vi "Main.vi"() -> ()   [LabVIEW 2017]
doc: "Use this template to build a simple state machine design pattern. Each state executes code and determines which state to transition to."
uses:
  Controls/Database_Array.ctl
  Controls/Encoding.ctl
  <userlib>/_OpenG.lib/array/array.llb/Search 1D Array (I32)__ogtk.vi
  <userlib>/_OpenG.lib/array/array.llb/Index 1D Array Elements (Variant)__ogtk.vi
  Controls/State.ctl
  Controls/Data.ctl
panel:
  out "Error (out)":errorcluster
  out "Parameter Array":T1[](array[typedef])
  out "HW File":string
  out "Param File":string
  in  "Core ID":i32=-1
  in  "Core Name":string="CoreName"
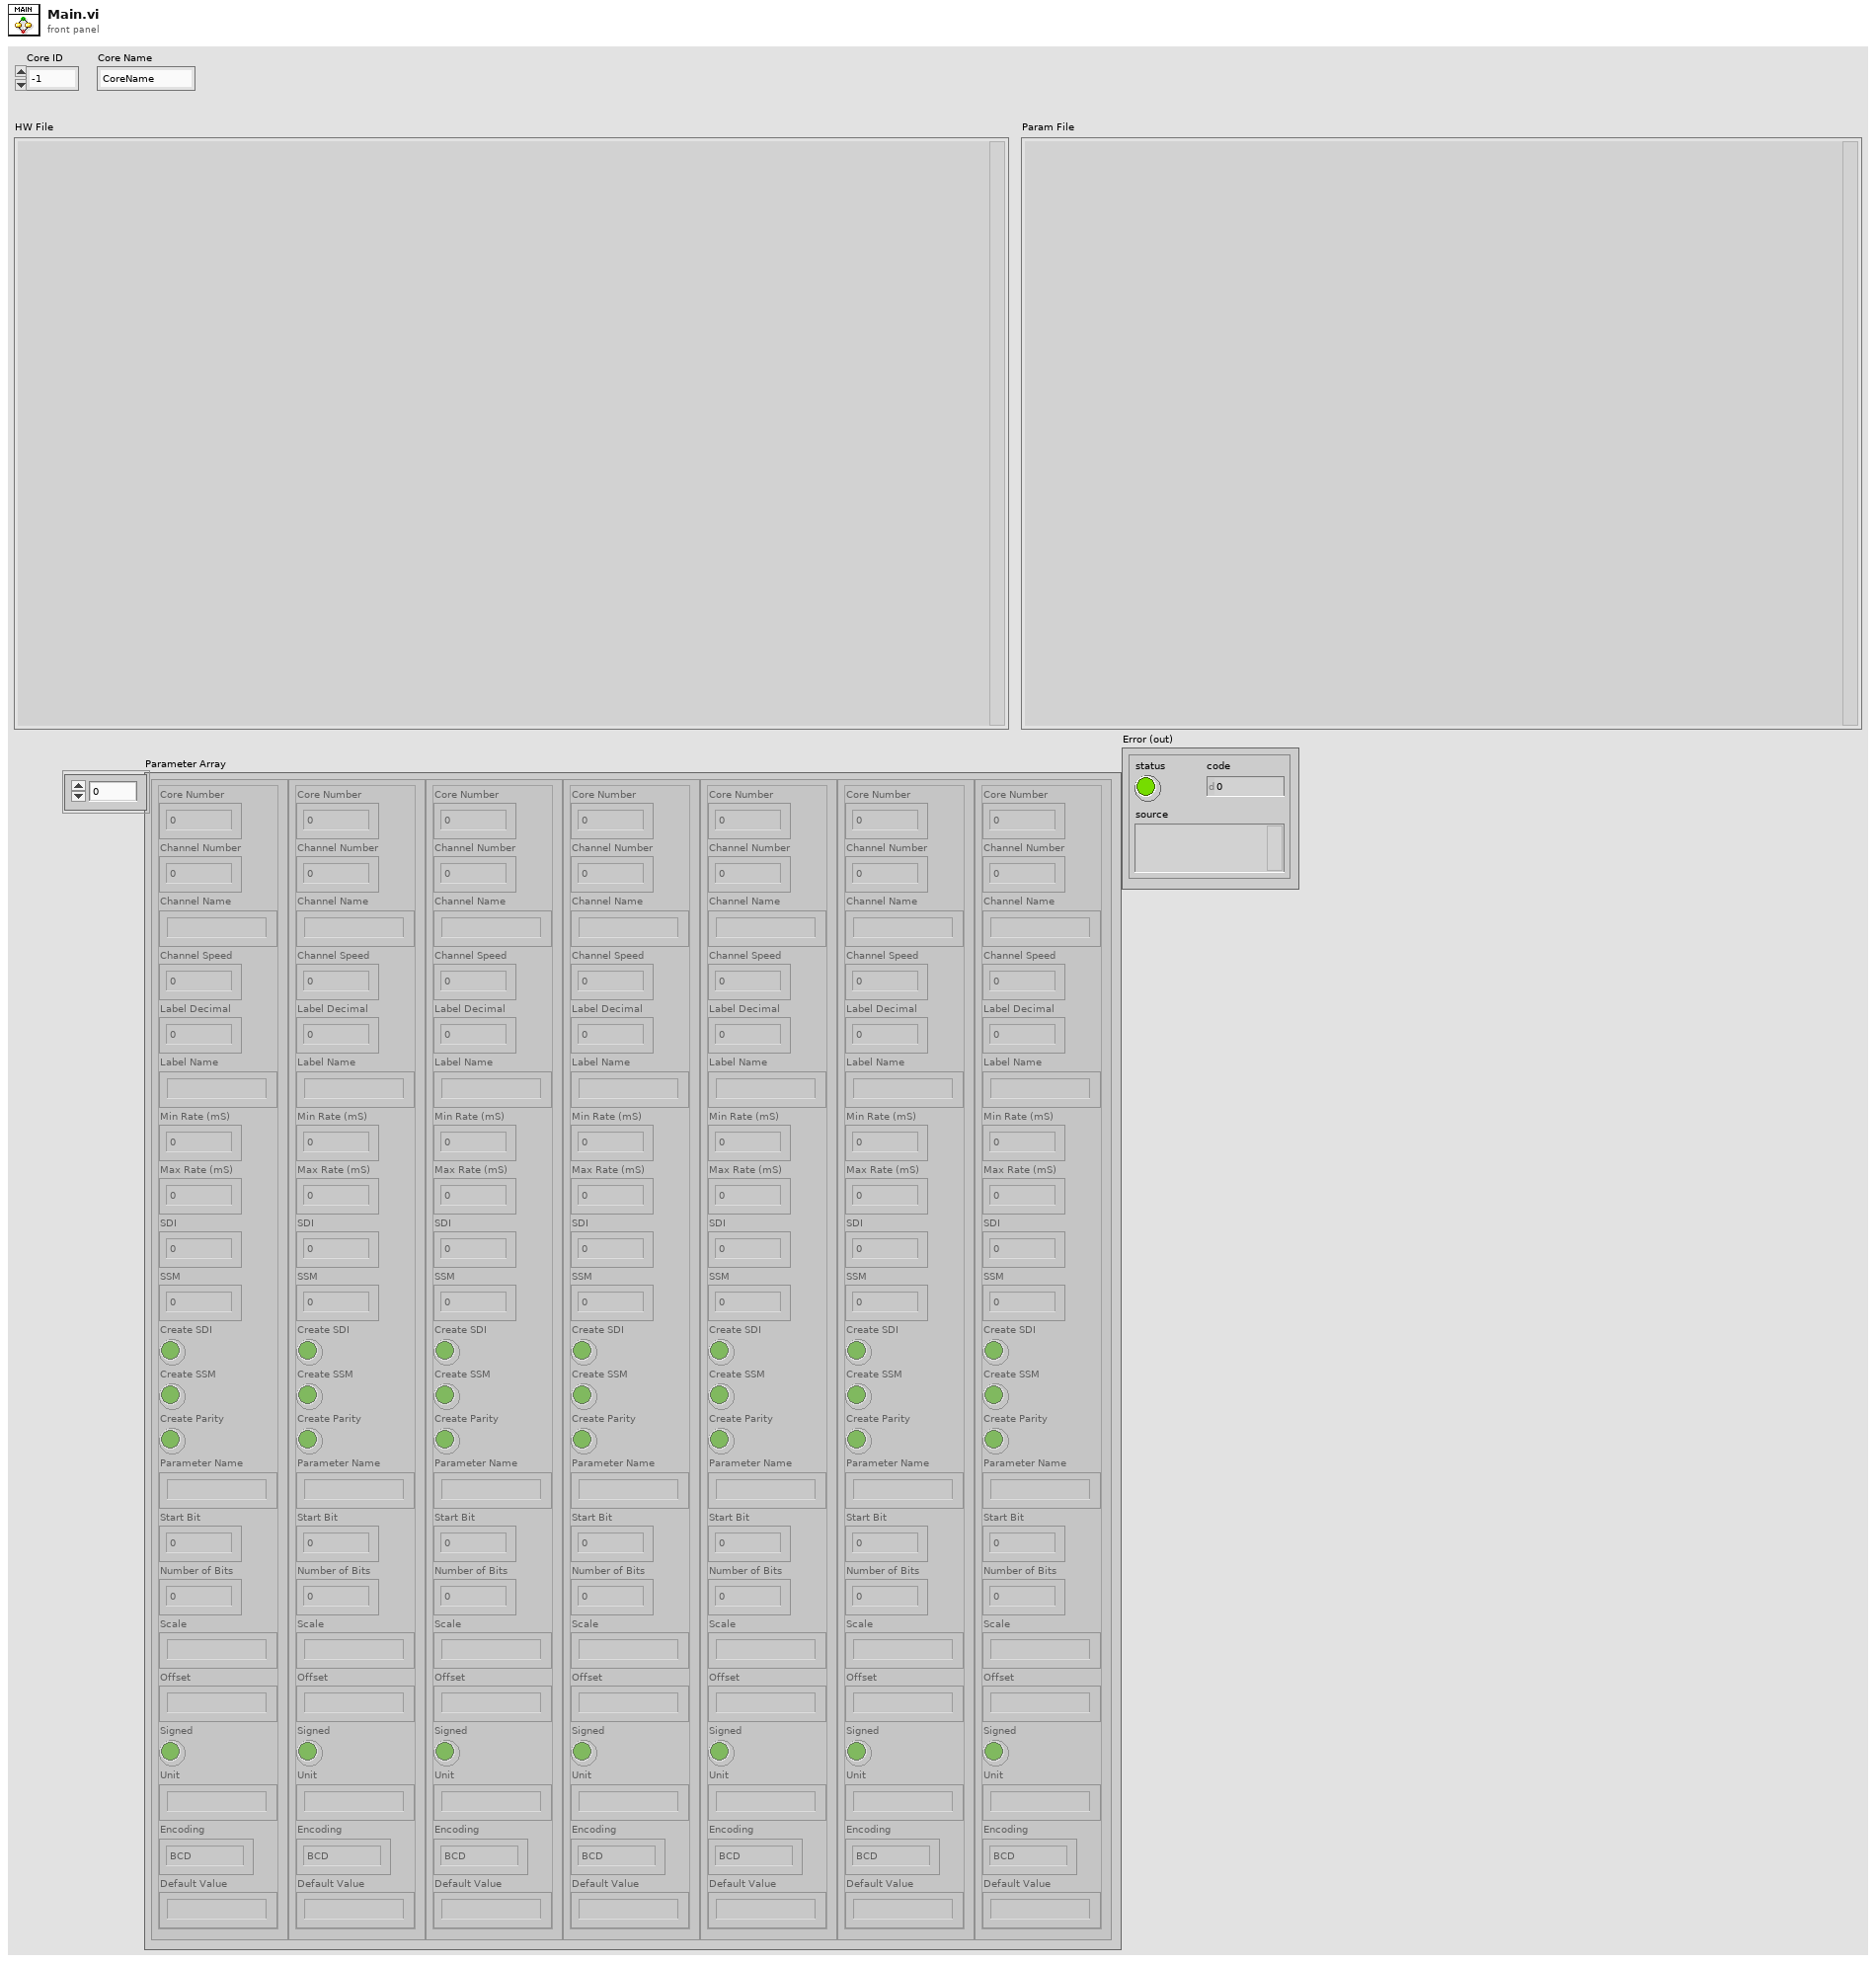
[diagram p1: front panel]
types:
  T1 = typedef "Database_Array.ctl" = cluster{"Core Number":i32, "Channel Number":i32, "Channel Name":string, "Channel Speed":i32, "Label Decimal":i32, "Label Name":string, "Min Rate (mS)":i32, "Max Rate (mS)":i32, "SDI":i32, "SSM":i32, "Create SDI":bool, "Create SSM":bool, "Create Parity":bool, "Parameter Name":string, "Start Bit":i32, "Number of Bits":i32, "Scale":string, "Offset":string, "Signed":bool, "Unit":string, "Encoding":T2, "Default Value":string}
  T2 = typedef "Encoding.ctl" = enum16{"BCD", "BNR", "Discrete"}
  T3 = typedef "Data.ctl" = cluster{"HW XML":string, "Parameter XML":string, "Database []":T1}
  T4 = typedef "State.ctl" = enum16{"Initialize", "Wait for Event", "HW XML - Open", "HW XML - Rx", "HW XML - Tx", "HW XML - Close", "User State 2", "Exit"}
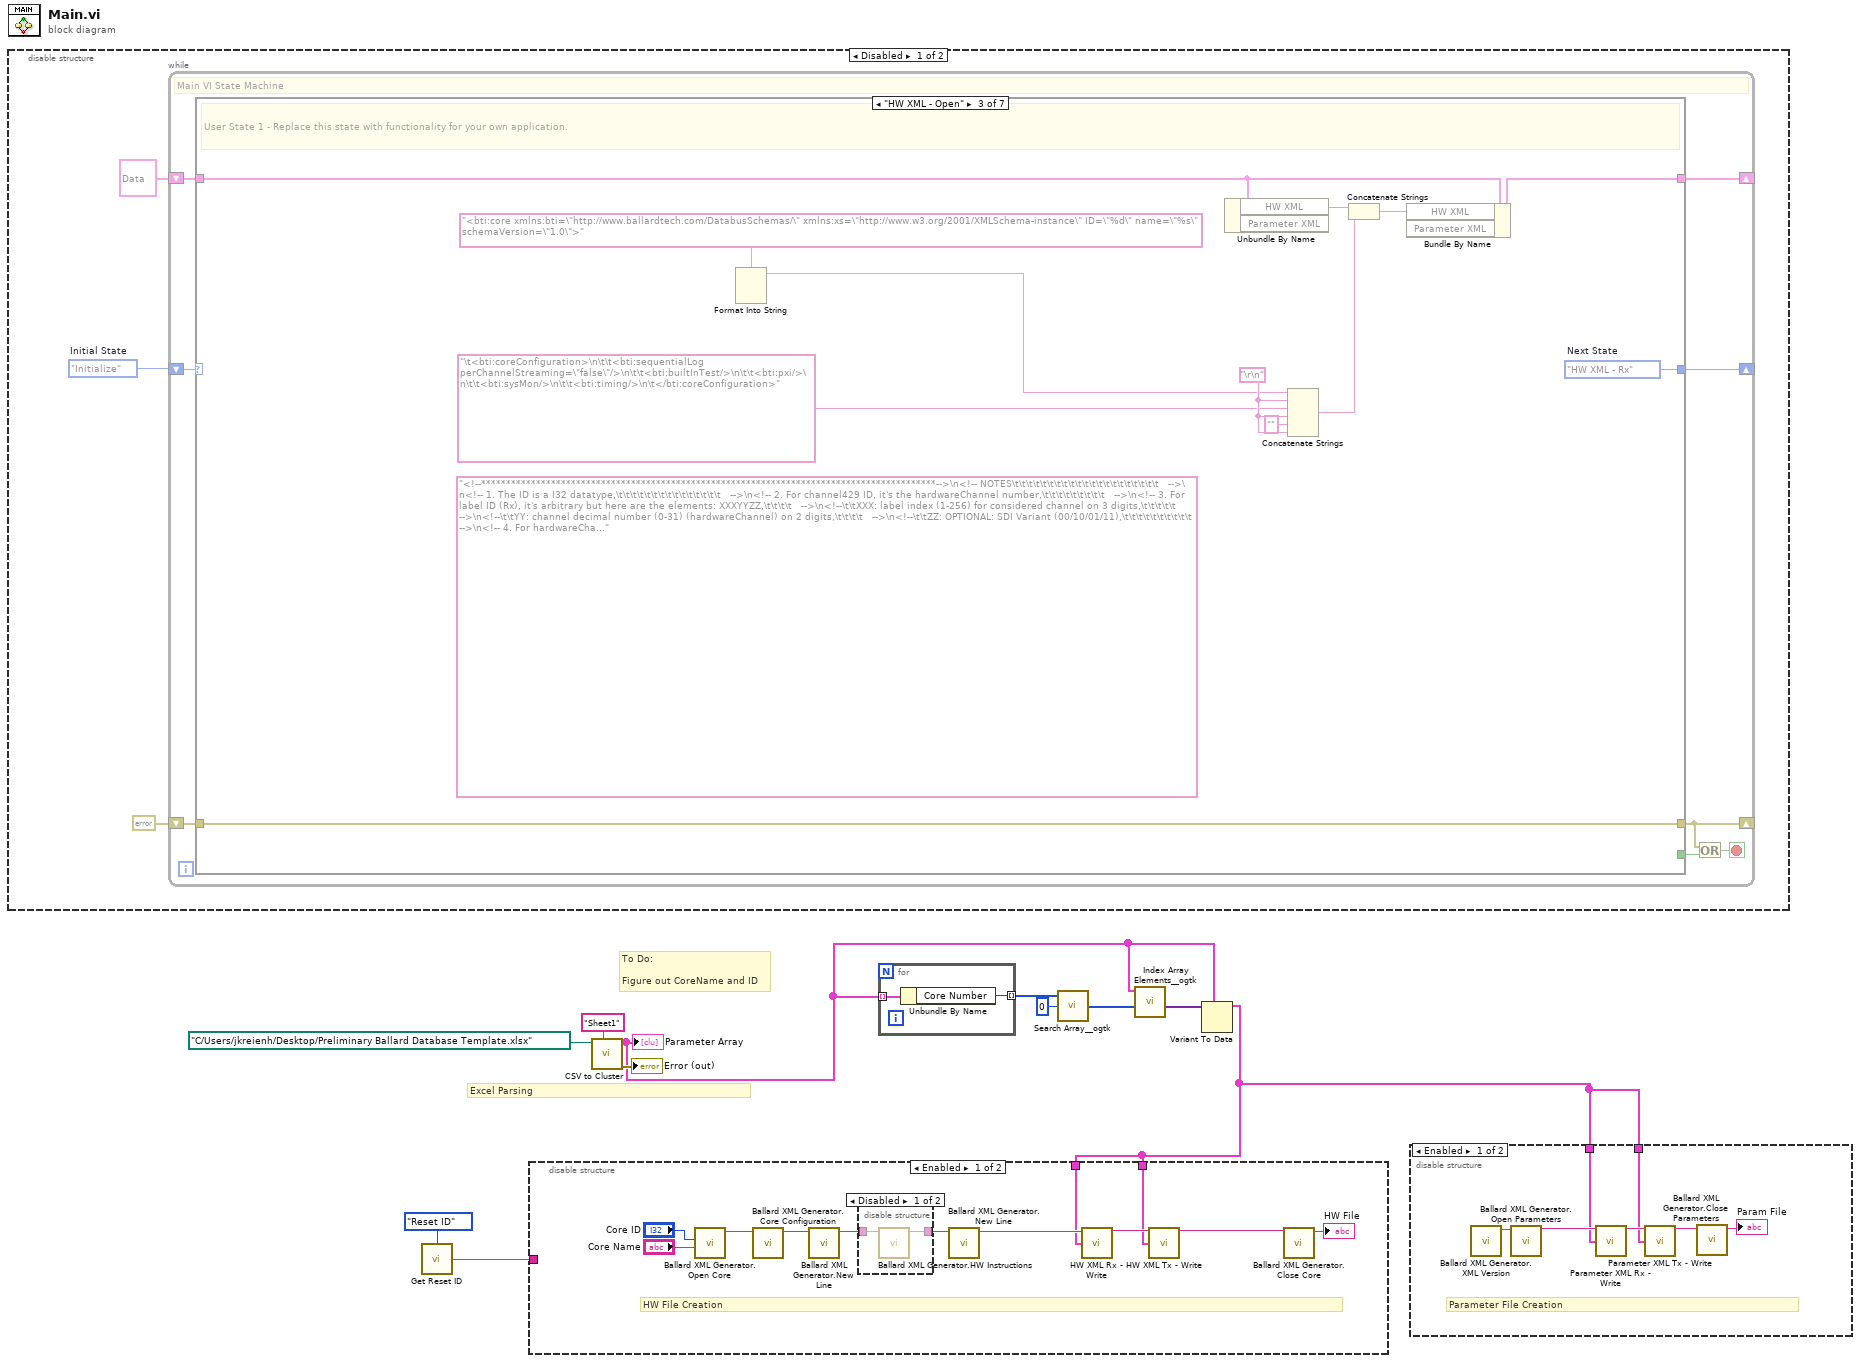
[diagram p0: block diagram]
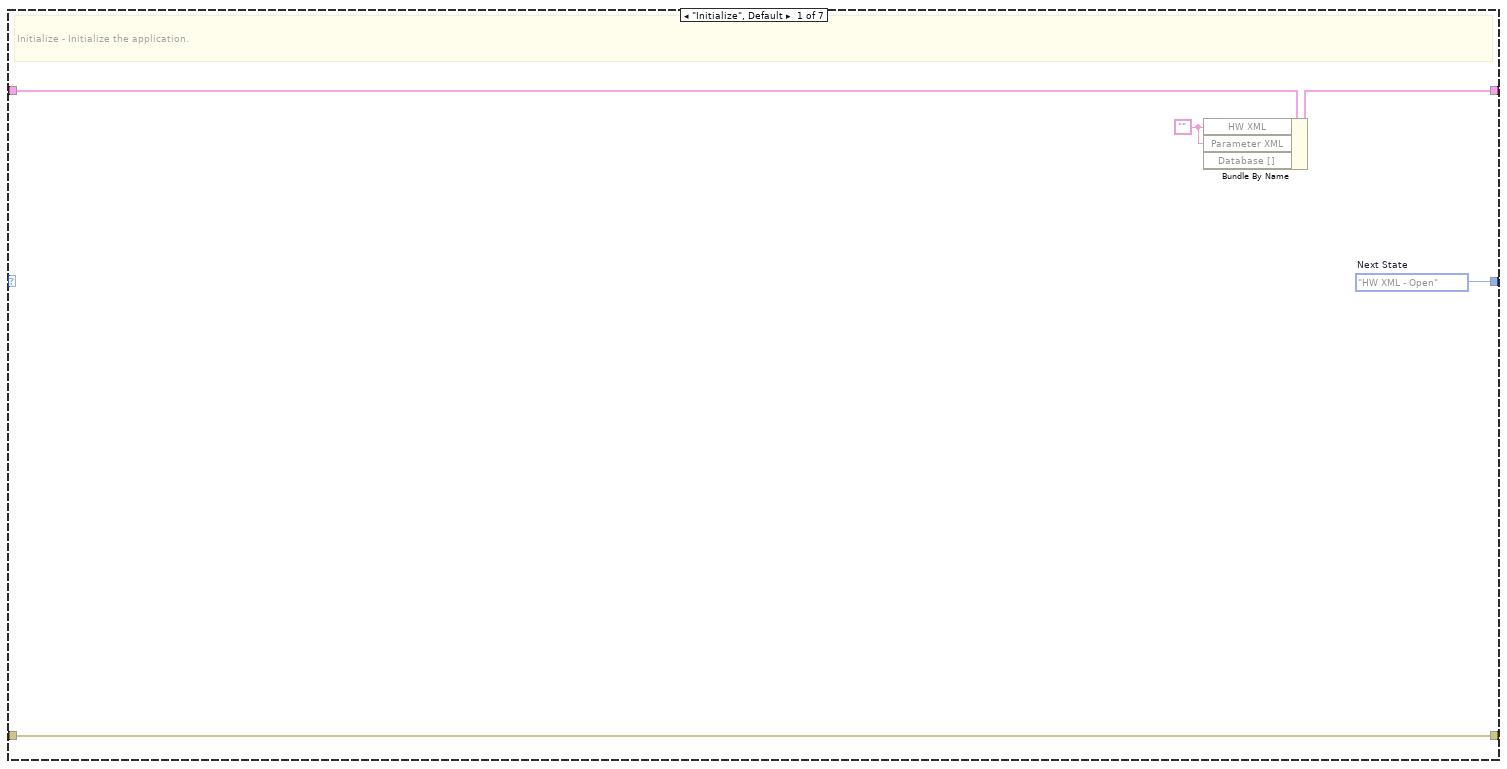
[diagram p5: hidden frame]
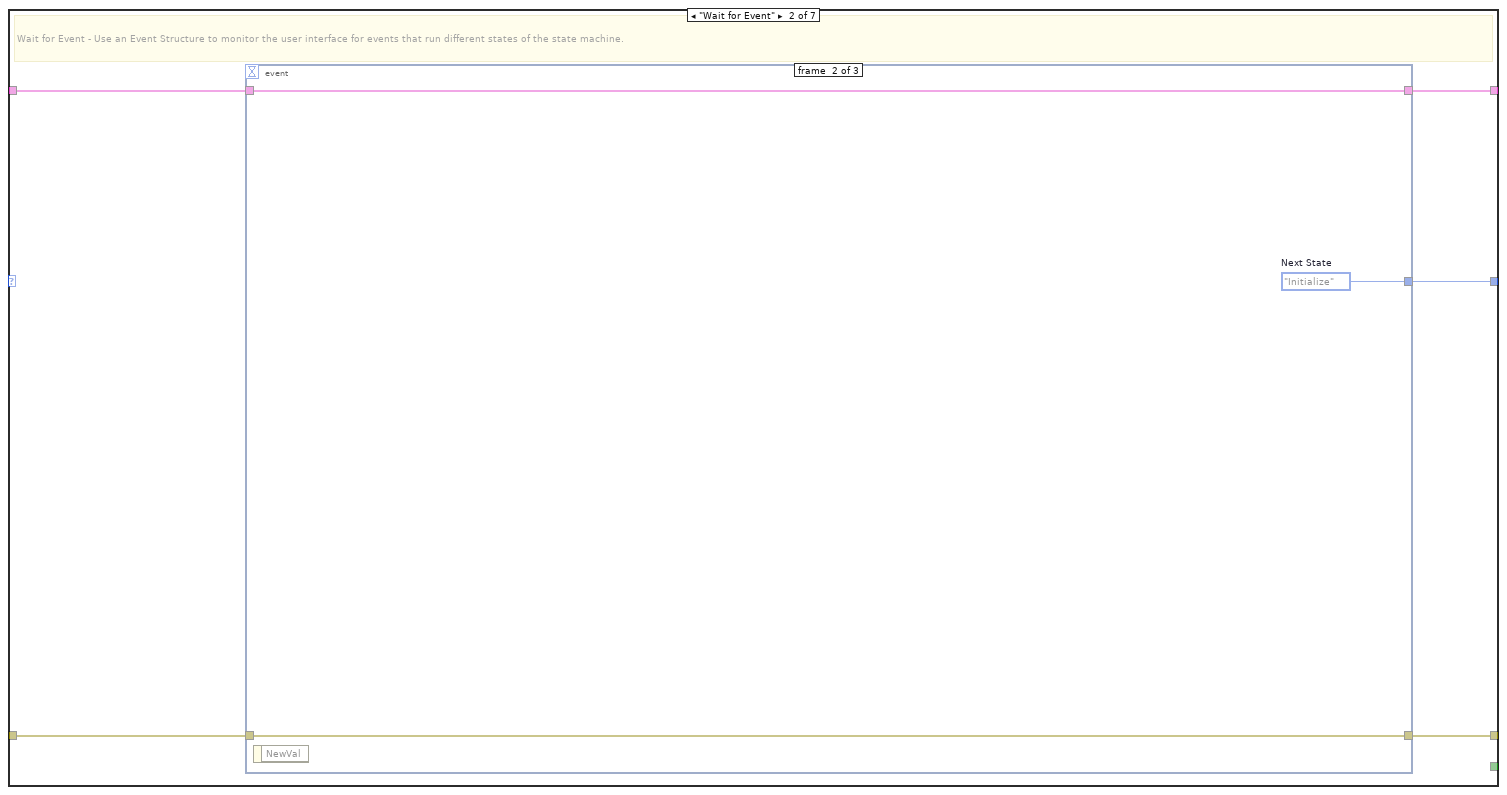
[diagram p6: hidden frame]
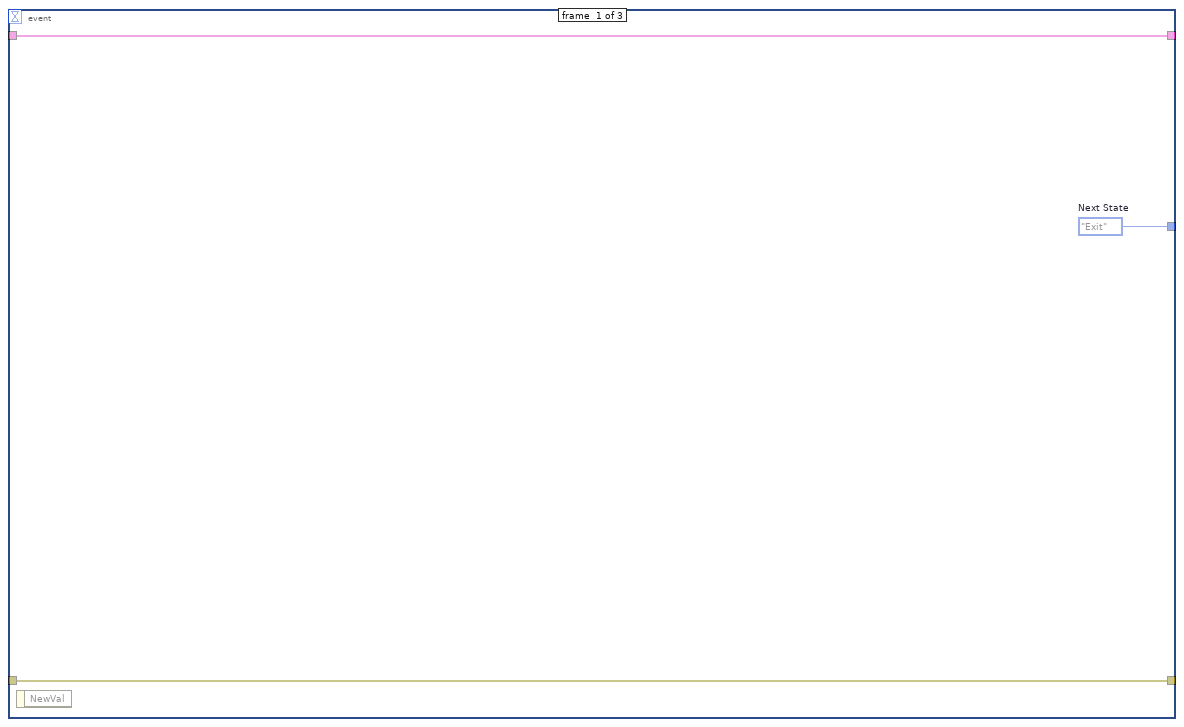
[diagram p7: hidden frame]
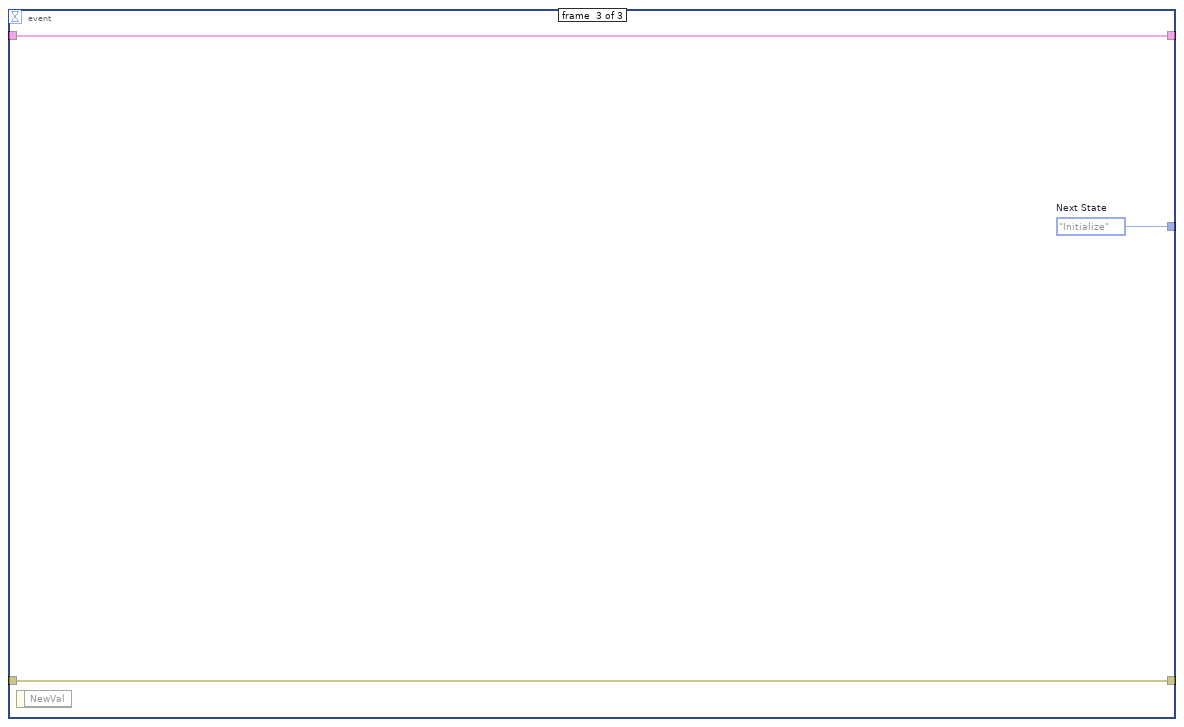
[diagram p8: hidden frame]
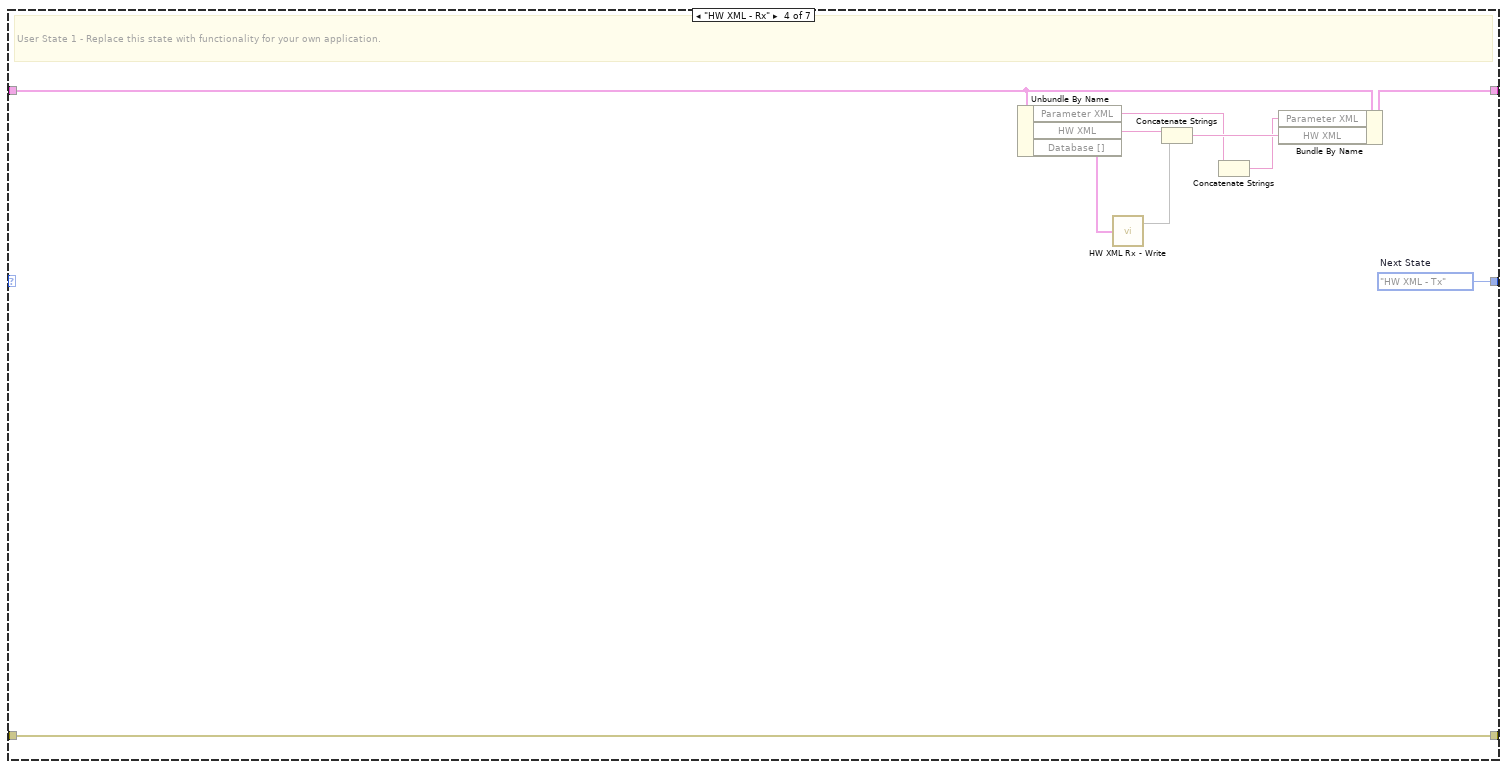
[diagram p9: hidden frame]
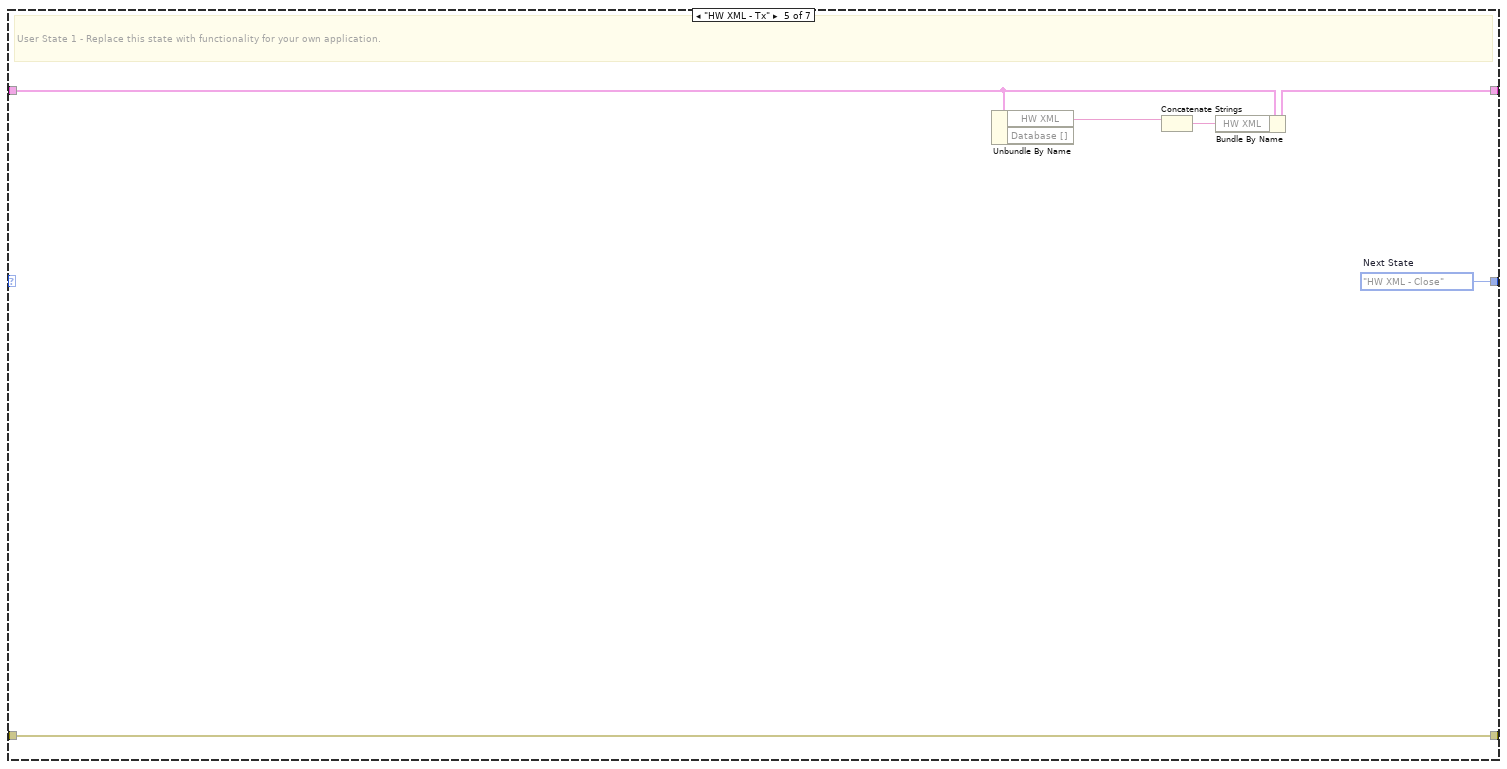
[diagram p10: hidden frame]
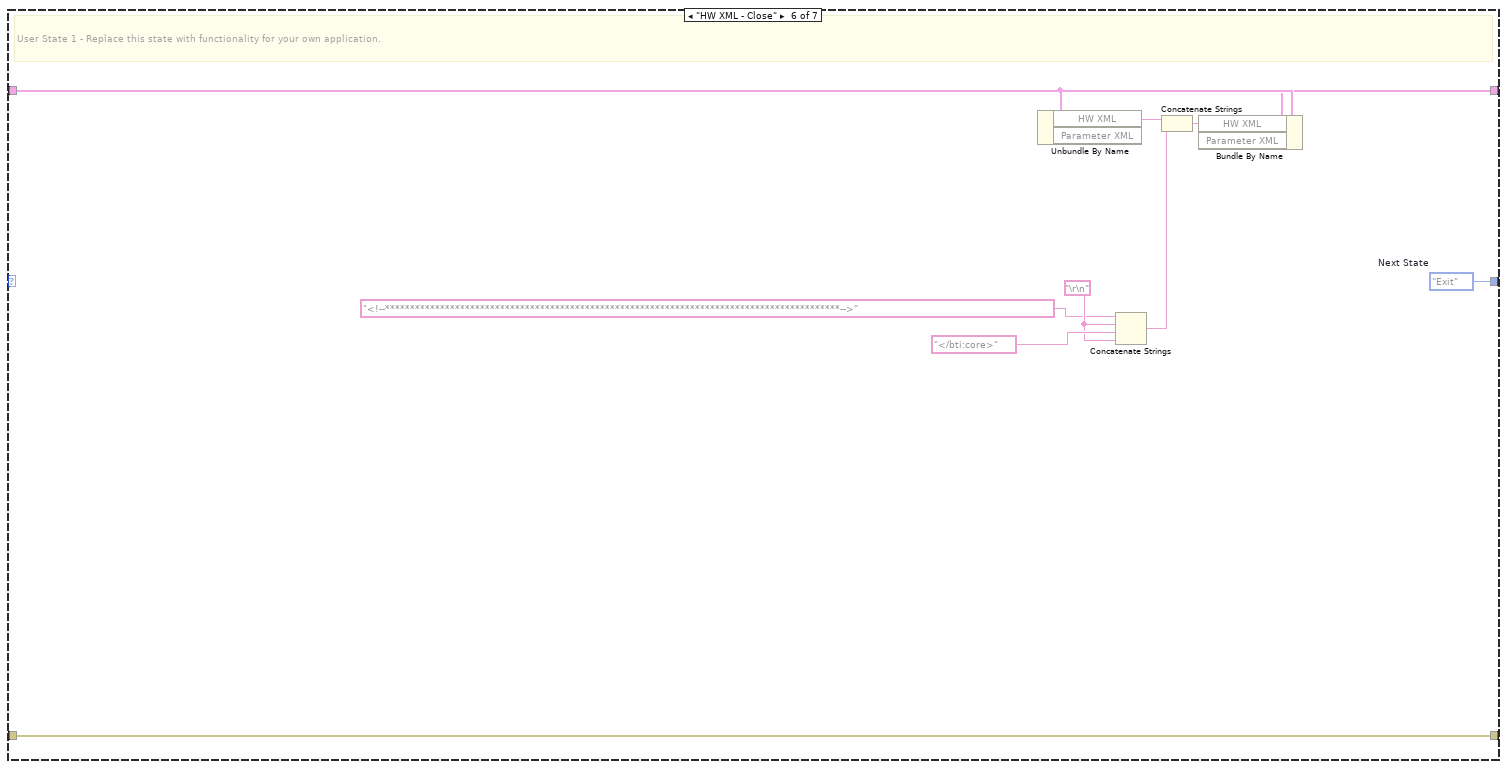
[diagram p11: hidden frame]
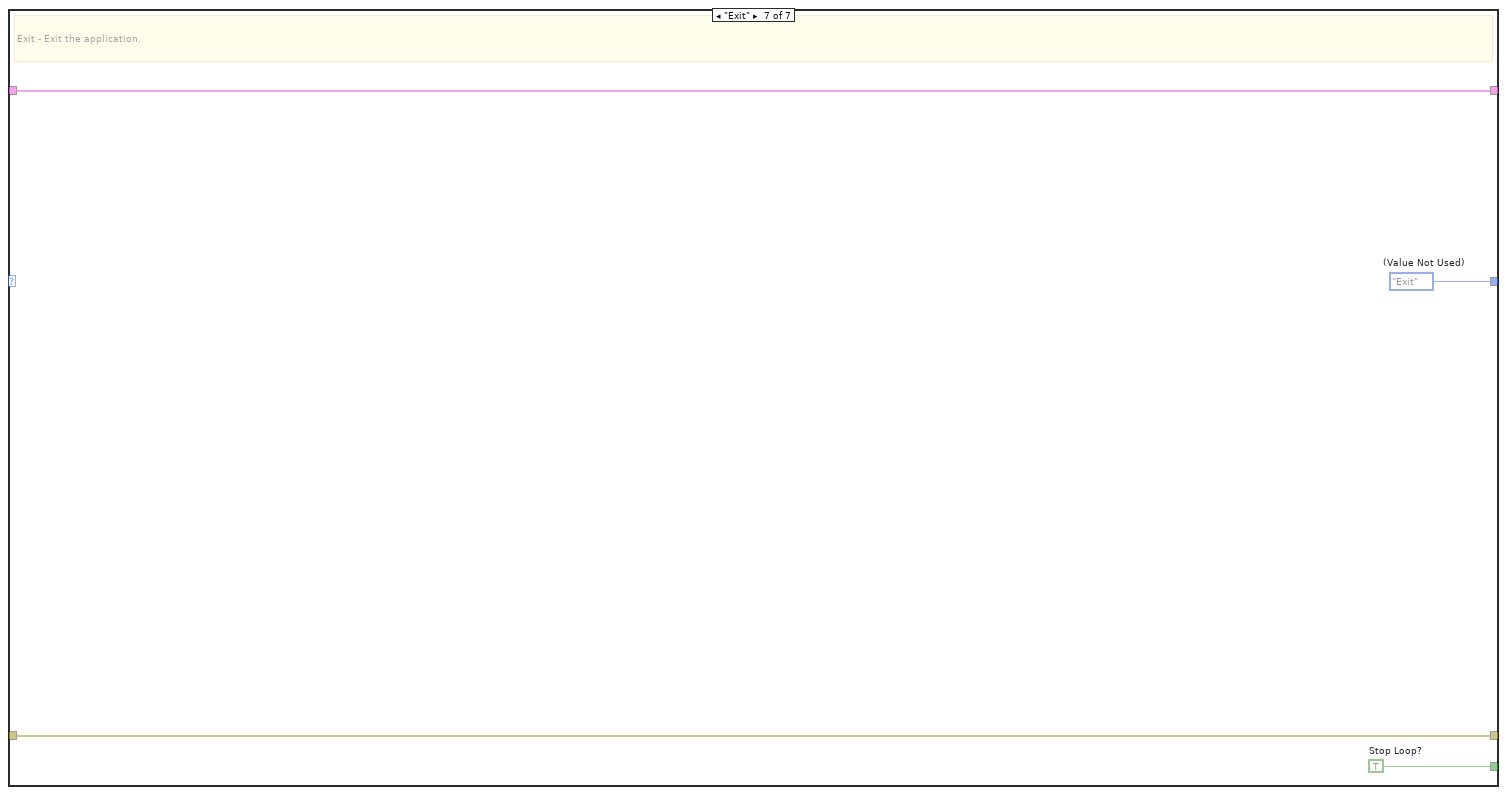
[diagram p12: hidden frame]
diagram:
  # "Excel Parsing"
  # "To Do:\n\nFigure out CoreName and ID"
  n1 = disable-structure shown="Disabled" {
    frame Disabled {
      w14 = State."Initialize"  # Initial State
      n2 = while {
        shift-right: [w21] -> _
        shift-left: w14 -> [w22]
        shift-right: [w19] -> _
        shift-left: T3 {"HW XML"="", "Parameter XML"="", "Database []"={"Core Number"=0, "Channel Number"=0, "Channel Name"="", "Channel Speed"=0, "Label Decimal"=0, "Label Name"="", "Min Rate (mS)"=0, "Max Rate (mS)"=0, "SDI"=0, "SSM"=0, "Create SDI"=FALSE, "Create SSM"=FALSE, "Create Parity"=FALSE, "Parameter Name"="", "Start Bit"=0, "Number of Bits"=0, "Scale"="", "Offset"="", "Signed"=FALSE, "Unit"="", "Encoding"=enum."BCD", "Default Value"=""}} ("Data") -> [w20]
        shift-right: [w15] -> _
        shift-left: errorcluster {"status"=FALSE, "code"=0, "source"=""} ("error constant") -> [w18]
        stop <- w16 stop-if-true
        # "Main VI State Machine"
        n3 = case shown="\"HW XML - Open\"" w22 {
          tunnel: [w28 w33 w57 w68 w76 w87 w91] -> w21
          tunnel: [_ _ _ _ _ _ w89] -> w17
          tunnel: w20 -> [w26 w32 w48 w65 w73 w84 w90]
          tunnel: [w25 w31 w46 w63 w71 w82 w90] -> w19
          tunnel: w18 -> [w27 w30 w56 w67 w75 w86 w88]
          tunnel: [w27 w29 w56 w67 w75 w86 w88] -> w15
          frame "Initialize", Default {
            w24 = ""
            w28 = State."HW XML - Open"  # Next State
            # "Initialize - Initialize the application."
            n4 = Bundle By Name(cluster=w26, "HW XML"=w24, "Parameter XML"=w24) -> (w25:T3, "Database []"=w23:T1)
          }
          frame "Wait for Event" {
            # "Wait for Event - Use an Event Structure to monitor the user interface for events that run different states of the state machine."
            n5 = event {
              selector: _ -> [_ _ _]
              dyn-events: _ -> [_ _ _]
              timeout: _ -> [_ _ _]
              tunnel: [w36 w39 w42] -> w33
              tunnel: w32 -> [w35 w37 w40]
              tunnel: [w35 w37 w40] -> w31
              tunnel: w30 -> [w34 w38 w41]
              tunnel: [w34 w38 w41] -> w29
              event #0 {
                w36 = State."Exit"  # Next State
                n6 = event-data() -> ()  [unwired: 1 in, 1 out]
              }
              event #1 {
                w39 = State."Initialize"  # Next State
                n7 = event-data() -> ()  [unwired: 1 in, 1 out]
              }
              event #2 {
                w42 = State."Initialize"  # Next State
                n8 = event-data() -> ()  [unwired: 1 in, 1 out]
              }
            }
          }
          frame "HW XML - Open" {
            (unwired) "<!--*******************************************************************************************-->\n<!-- NOTES\t\t\t\t\t\t\t\t\t\t\t\t\t\t\t\t\t\t\t\t\t   -->\n<!-- 1. The ID is a I32 datatype,\t\t\t\t\t\t\t\t\t\t\t\t\t\t\t   -->\n<!-- 2. For channel429 ID, it's the hardwareChannel number,\t\t\t\t\t\t\t\t\t   -->\n<!-- 3. For label ID (Rx), it's arbitrary but here are the elements: XXXYYZZ,\t\t\t\t   -->\n<!--\t\tXXX: label index (1-256) for considered channel on 3 digits,\t\t\t\t\t   -->\n<!--\t\tYY: channel decimal number (0-31) (hardwareChannel) on 2 digits,\t\t\t\t   -->\n<!--\t\tZZ: OPTIONAL: SDI Variant (00/10/01/11),\t\t\t\t\t\t\t\t\t\t   -->\n<!-- 4. For hardwareChannel numbering, for a core with 16 (Rx/Tx) Channels, Rx Channels are\t   -->\n<!-- numbered between 0 and 15, Tx Channels are numbered between 16 and 31. Physically, for    -->\n<!-- instance, hardwareChannel 1 and 17 are the same but the direction is different.\t\t   -->\n<!-- 5. For message ID (Tx), it's arbitrary but here are the elements: XXXYYZZZ,\t\t\t   -->\n<!--\t\tXXX`: label index (1-256) for considered channel on 3 digits,\t\t\t\t\t   -->\n<!--\t\tYY: channel decimal number (0-31) (hardwareChannel) on 2 digits,\t\t\t\t   -->\n<!-- 6. For messageBuffer ID (Tx), it's arbitrary but here are the elements: XXXYYZZZ,\t\t   -->\n<!--\t\tXXX`: label index (1-999) for considered channel on 3 digits,\t\t\t\t\t   -->\n<!--\t\tYY: channel decimal number (0-31) (hardwareChannel) on 2 digits,\t\t\t\t   -->\n<!--\t\tZZZ: messageBuffer Index on 3 digits (1-999),\t\t\t\t\t\t\t\t\t   -->\n<!-- 7. For Rx Channels, it's important to list ALL labels physically present on the Channel   -->\n<!--    and, for each, set \"monitor\" element to true or false.\t\t\t\t\t\t\t\t   -->\n<!--*******************************************************************************************-->"
            w53 = "\r\n"
            w57 = State."HW XML - Rx"  # Next State
            # "User State 1 - Replace this state with functionality for your own application."
            n9 = Format Into String(format string="<bti:core xmlns:bti=\"http://www.ballardtech.com/DatabusSchemas/\" xmlns:xs=\"http://www.w3.org/2001/XMLSchema-instance\" ID=\"%d\" name=\"%s\" schemaVersion=\"1.0\">") -> (resulting string=w52:string, w54:i32, w55:string)  [unwired: 2 in, 1 out]
            n10 = Unbundle By Name(w48) -> ("HW XML"=w50:string, "Parameter XML"=w43:string)
            n11 = Concatenate Strings(w52, w53, "\t<bti:coreConfiguration>\n\t\t<bti:sequentialLog perChannelStreaming=\"false\"/>\n\t\t<bti:builtInTest/>\n\t\t<bti:pxi/>\n\t\t<bti:sysMon/>\n\t\t<bti:timing/>\n\t</bti:coreConfiguration>" ("string"), w53, "" ("string"), w53) -> (w49:string)
            n12 = Concatenate Strings(w50, w49) -> (w47:string)
            n13 = Bundle By Name(cluster=w48, "HW XML"=w47) -> (w46:T3)  [unwired: 1 in]
          }
          frame "HW XML - Rx" {
            w68 = State."HW XML - Tx"  # Next State
            # "User State 1 - Replace this state with functionality for your own application."
            n14 = Unbundle By Name(w65) -> ("Parameter XML"=w59:string, "HW XML"=w66:string, "Database []"=w61:T1)
            n15 = call "HW XML Rx - Write.vi"("Parameter Array"=w61) -> (8:w62)  [unwired: 13 in, 1 out]
            n16 = Concatenate Strings(w66, w62) -> (w64:string)
            n17 = Concatenate Strings(w59) -> (w60:string, w58:string)
            n18 = Bundle By Name(cluster=w65, "Parameter XML"=w60, "HW XML"=w64) -> (w63:T3)
          }
          frame "HW XML - Tx" {
            w76 = State."HW XML - Close"  # Next State
            # "User State 1 - Replace this state with functionality for your own application."
            n19 = Unbundle By Name(w73) -> ("HW XML"=w74:string, "Database []"=w69:T1)
            n20 = Concatenate Strings(w74) -> (w72:string, w70:string)
            n21 = Bundle By Name(cluster=w73, "HW XML"=w72) -> (w71:T3)
          }
          frame "HW XML - Close" {
            w80 = "\r\n"
            w87 = State."Exit"  # Next State
            # "User State 1 - Replace this state with functionality for your own application."
            n22 = Unbundle By Name(w84) -> ("HW XML"=w85:string, "Parameter XML"=w77:string)
            n23 = Concatenate Strings("<!--*******************************************************************************************-->", w80, "</bti:core>" ("string"), w80) -> (w79:string)
            n24 = Concatenate Strings(w85, w79) -> (w83:string)
            n25 = Bundle By Name(cluster=w84, "HW XML"=w83) -> (w82:T3)  [unwired: 1 in]
          }
          frame "Exit" {
            w89 = TRUE  # Stop Loop?
            w91 = State."Exit"  # (Value Not Used)
            # "Exit - Exit the application."
          }
        }
        n26 = Or(x=w15, y=w17) -> (x .or. y?=w16:bool)
      }
    }
    frame Enabled {
    }
  }
  n27 = call "Get Reset ID.vi"("Function"=enum16{"Get ID", "Reset ID"}."Reset ID") -> ("ID"=w1:string)  [unwired: 14 in]
  n28 = call "CSV to Cluster.vi"("Excel._SheetName"="Sheet1", "file path (dialog if empty)"=path "C:/Users/jkreienh/Desktop/Preliminary Ballard Database Template.xlsx") -> ("Error (out)"=→"Error (out)":errorcluster, "Parameter Array"=w4:T1[])  [unwired: 8 in]
  "Parameter Array" <- w4
  n29 = for {
    tunnel: w4 -> [w93] mode=indexing
    tunnel: [w92] -> w8 mode=indexing
    n30 = Unbundle By Name(w93) -> ("Core Number"=w92:i32)
  }
  n31 = call-poly <userlib>:"Search Array__ogtk.vi"("Array"=w8, "Element Data"=0) -> ("Indices of Elements"=w6:i32[])  [unwired: 7 in]
  n32 = call-poly <userlib>:"Index Array Elements__ogtk.vi"("indices"=w6, "array"=w4) -> ("elements"=w5:variant[])  [unwired: 9 in]
  n33 = Variant To Data(type=w4, Variant=w5) -> (data=w3:T1[])  [unwired: 1 in, 1 out]
  n34 = disable-structure shown="Enabled" {
    disable-tunnel: w3 -> [w96 _]
    disable-tunnel: w3 -> [w95 _]
    disable-tunnel: w1 -> [_ _]
    frame Enabled {
      # "HW File Creation"
      n35 = call "Ballard XML Generator.Open Core.vi"("name"="Core Name", "id"="Core ID") -> ("string out"=w105:string)  [unwired: 9 in]
      n36 = call "Ballard XML Generator.Core Configuration.vi"("string in"=w105) -> ("string out"=w104:string)  [unwired: 10 in]
      n37 = call "Ballard XML Generator.New Line.vi"("string in"=w104) -> ("string out"=w103:string)  [unwired: 10 in]
      n38 = disable-structure shown="Disabled" {
        disable-tunnel: w103 -> [w107 w108]
        disable-tunnel: [w106 w108] -> w102
        frame Disabled {
          n39 = call "Ballard XML Generator.HW Instructions.vi"("string in"=w107) -> ("string out"=w106:string)  [unwired: 10 in]
        }
        frame Enabled {
        }
      }
      n40 = call "Ballard XML Generator.New Line.vi"("string in"=w102) -> ("string out"=w99:string)  [unwired: 10 in]
      n41 = call "HW XML Rx - Write.vi"("String (in)"=w99, "Parameter Array"=w96) -> ("String (out)"=w98:string)  [unwired: 13 in]
      n42 = call "HW XML Tx - Write.vi"("String (in)"=w98, "Parameter Array"=w95) -> ("String (out)"=w94:string)  [unwired: 13 in]
      n43 = call "Ballard XML Generator.Close Core.vi"("string in"=w94) -> ("string out"=→"HW File":string)  [unwired: 10 in]
    }
    frame Disabled {
    }
  }
  n44 = disable-structure shown="Enabled" {
    disable-tunnel: w3 -> [w110 _]
    disable-tunnel: w3 -> [w109 _]
    frame Enabled {
      # "Parameter File Creation"
      n45 = call "Ballard XML Generator.XML Version.vi"() -> ("string out"=w115:string)  [unwired: 11 in]
      n46 = call "Ballard XML Generator.Open Parameters.vi"("string in"=w115) -> ("string out"=w114:string)  [unwired: 10 in]
      n47 = call "Parameter XML Rx - Write.vi"("String (in)"=w114, "Parameter Array"=w110) -> ("String (out)"=w112:string)  [unwired: 13 in]
      n48 = call "Parameter XML Tx - Write.vi"("String (in)"=w112, "Parameter Array"=w109) -> ("String (out)"=w111:string)  [unwired: 13 in]
      n49 = call "Ballard XML Generator.Close Parameters.vi"("string in"=w111) -> ("string out"=→"Param File":string)  [unwired: 10 in]
    }
    frame Disabled {
    }
  }
